vi "DSF Mini Explorer.vi"(7 "Item Type":T1=enum."Setting", 8 "error in (no error)":errorcluster, 10 "Item ID":string, 11 "explorer data":T2) -> (0 "error out":errorcluster)   [LabVIEW 2017, in "DSF Mini Explorer.lvlib"]
uses:
  DSF Mini Explorer.lvlib
  Main VI/Application Data.ctl
  VeriStand/Data Sharing Custom Device/Source/DSF Core.lvlibp/Classes/Configuration/Configuration Session.lvclass
  Main VI/View Mode.ctl
  Item Tree/ID to Tree Items/Tree Item Type.ctl
  Item Tree/Create New Tree Item.vi
  VeriStand/Data Sharing Custom Device/Source/DSF Core.lvlibp/Classes/Configuration/Remove ID.vi
  VeriStand/Data Sharing Custom Device/Source/DSF Core.lvlibp/Classes/Configuration/Read Item.vi
  VeriStand/Data Sharing Custom Device/Source/DSF Core.lvlibp/Classes/Configuration/Read Plugin.vi
  VeriStand/Data Sharing Custom Device/Source/DSF Core.lvlibp/Classes/Configuration/Read Settings.vi
  VeriStand/Data Sharing Custom Device/Source/DSF Core.lvlibp/Classes/Configuration/Read Group.vi
  VeriStand/Data Sharing Custom Device/Source/DSF Core.lvlibp/Classes/Configuration/Read Transfer.vi
  VeriStand/Data Sharing Custom Device/Source/DSF Core.lvlibp/Classes/Configuration/Read Channel.vi
panel:
  in  "Item Tree":string(tree)
  in  "Value Tree":string(tree)
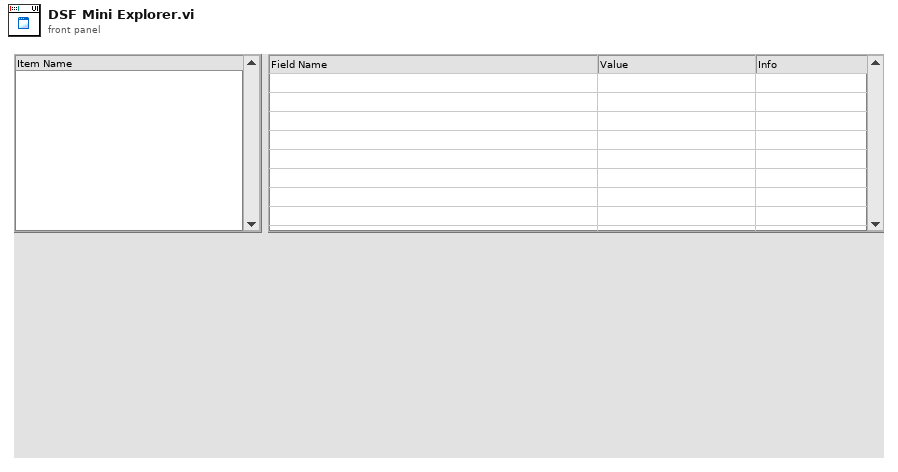
[diagram p1: front panel]
types:
  T1 = typedef "DSF Mini Explorer.lvlib/Tree Item Type.ctl" = enum16{"Plugin", "Group", "Transfer", "Channel", "Setting"}
  T2 = typedef "DSF Mini Explorer.lvlib/Application Data.ctl" = cluster{"Item Tree Control":refnum<vi>, "Value Tree Control":refnum<vi>, "DSF Refnum":refnum<class "Configuration Session.lvclass">, "Top-Level VI":refnum<vi>, "View State":T3}
  T3 = typedef "DSF Mini Explorer.lvlib/View Mode.ctl" = enum16{"Tree", "List"}
  T4 = typedef "DSF Mini Explorer.lvlib/Tree Item.ctl" = cluster{"Left Cell String":string, "Child Text":string[], "Child Tag":string, "Glyph Index":i32}
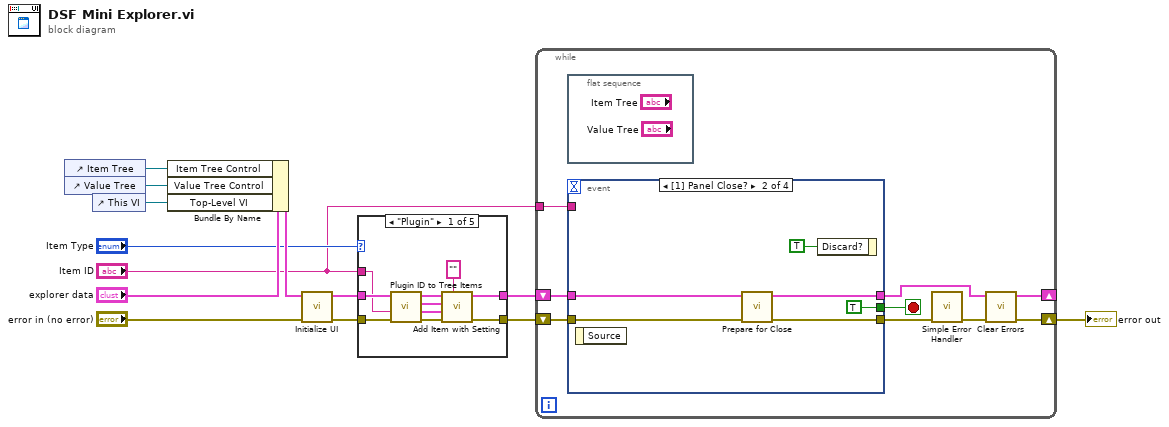
[diagram p0: block diagram]
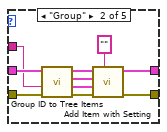
[diagram p2: hidden frame]
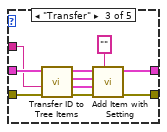
[diagram p3: hidden frame]
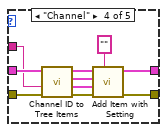
[diagram p4: hidden frame]
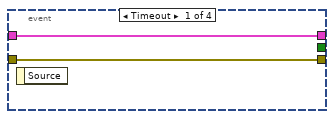
[diagram p6: hidden frame]
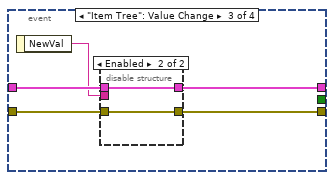
[diagram p7: hidden frame]
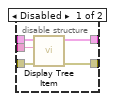
[diagram p8: hidden frame]
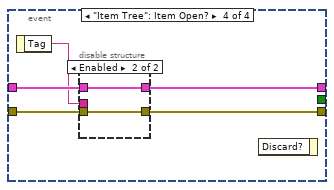
[diagram p9: hidden frame]
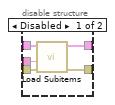
[diagram p10: hidden frame]
diagram:
  n1 = control-ref of="Item Tree"() -> (w9:refnum<vi>)
  n2 = control-ref of="Value Tree"() -> (w10:refnum<vi>)
  n3 = control-ref of="This VI"() -> (w2:refnum<vi>)
  n4 = Bundle By Name(cluster="explorer data", "Item Tree Control"=w9, "Value Tree Control"=w10, "Top-Level VI"=w2) -> (w12:T2)
  n5 = call "Initialize UI.vi"("error in (no error)"="error in (no error)", "Application Data in"=w12) -> ("error out"=w6:errorcluster, "Application Data out"=w7:T2)  [unwired: 8 in]
  n6 = case shown="\"Plugin\"" "Item Type" {
    tunnel: w7 -> [w23 w29 w40 w47 w55]
    tunnel: w6 -> [w22 w30 w38 w48 w54]
    tunnel: [w17 w32 w42 w52 w54] -> w5
    tunnel: [w18 w33 w43 w53 w55] -> w4
    tunnel: "Item ID" -> [w21 w24 w37 w46 _]
    frame "Plugin" {
      n7 = call "Plugin ID to Tree Items.vi"("error in (no error)"=w22, "Plugin ID"=w21, "Application Data in"=w23) -> ("error out"=w19:errorcluster, "Settings"=w15:T4, "Item"=w16:T4, "Application Data out"=w20:T2)  [unwired: 5 in]
      n8 = call "Add Item with Setting.vi"("Parent Tag"="", "error in (no error)"=w19, "Setting"=w15, "Item"=w16, "Application Data in"=w20) -> ("error out"=w17:errorcluster, "Application Data out"=w18:T2)  [unwired: 4 in, 1 out]
    }
    frame "Group" {
      n9 = call "Group ID to Tree Items.vi"("error in (no error)"=w30, "Group ID"=w24, "Application Data in"=w29) -> ("error out"=w27:errorcluster, "Settings"=w25:T4, "Item"=w26:T4, "Application Data out"=w28:T2)  [unwired: 5 in]
      n10 = call "Add Item with Setting.vi"("Parent Tag"="", "error in (no error)"=w27, "Setting"=w25, "Item"=w26, "Application Data in"=w28) -> ("error out"=w32:errorcluster, "Application Data out"=w33:T2)  [unwired: 4 in, 1 out]
    }
    frame "Transfer" {
      n11 = call "Transfer ID to Tree Items.vi"("error in (no error)"=w38, "Transfer ID"=w37, "Application Data in"=w40) -> ("error out"=w36:errorcluster, "Settings"=w35:T4, "Item"=w34:T4, "Application Data out"=w39:T2)  [unwired: 5 in]
      n12 = call "Add Item with Setting.vi"("Parent Tag"="", "error in (no error)"=w36, "Setting"=w35, "Item"=w34, "Application Data in"=w39) -> ("error out"=w42:errorcluster, "Application Data out"=w43:T2)  [unwired: 4 in, 1 out]
    }
    frame "Channel" {
      n13 = call "Channel ID to Tree Items.vi"("error in (no error)"=w48, "Channel ID"=w46, "Application Data in"=w47) -> ("error out"=w49:errorcluster, "Settings"=w44:T4, "Item"=w45:T4, "Application Data out"=w50:T2)  [unwired: 5 in]
      n14 = call "Add Item with Setting.vi"("Parent Tag"="", "error in (no error)"=w49, "Setting"=w44, "Item"=w45, "Application Data in"=w50) -> ("error out"=w52:errorcluster, "Application Data out"=w53:T2)  [unwired: 4 in, 1 out]
    }
    frame "Setting" {
    }
  }
  n15 = while {
    shift-right: [w57] -> w13
    shift-left: w5 -> [w62]
    shift-right: [w58] -> _
    shift-left: w4 -> [w59]
    tunnel: "Item ID" -> [w56]
    stop <- w63 stop-if-true
    n16 = flat-sequence {
      frame #0 {
      }
    }
    n17 = event shown="[1] Panel Close?" {
      selector: _ -> [_ _ _ _]
      dyn-events: _ -> [_ _ _ _]
      timeout: _ -> [_ _ _ _]
      tunnel: [_ TRUE _ _] -> w63
      tunnel: w62 -> [w65 w70 w76 w88]
      tunnel: [w65 w67 w75 w87] -> w60
      tunnel: w59 -> [w64 w68 w73 w86]
      tunnel: [w64 w66 w74 w85] -> w58
      tunnel: w56 -> [_ _ _ _]
      event Timeout {
        n18 = event-data() -> ()  [unwired: 1 in, 1 out]
      }
      event Panel Close? {
        n19 = event-data() -> ()  [unwired: 1 in, 1 out]
        n20 = call "Prepare for Close.vi"("error in (no error)"=w70, "Application Data in"=w68) -> ("error out"=w67:errorcluster, "Application Data out"=w66:T2)  [unwired: 8 in]
        n21 = event-data("Discard?"=TRUE) -> ()  [unwired: 1 in, 1 out]
      }
      event "Item Tree": Value Change {
        n22 = event-data() -> ("NewVal"=w72:string)  [unwired: 1 in]
        n23 = disable-structure shown="Enabled" {
          disable-tunnel: w76 -> [w81 w82]
          disable-tunnel: [w80 w82] -> w75
          disable-tunnel: [w79 w83] -> w74
          disable-tunnel: w73 -> [w78 w83]
          disable-tunnel: w72 -> [w77 _]
          frame Disabled {
            n24 = call "Display Tree Item.vi"("error in (no error)"=w81, "Tag"=w77, "Application Data in"=w78) -> ("error out"=w80:errorcluster, "Application Data out"=w79:T2)  [unwired: 7 in]
          }
          frame Enabled {
          }
        }
      }
      event "Item Tree": Item Open? {
        n25 = event-data() -> ("Tag"=w84:string)  [unwired: 1 in]
        n26 = disable-structure shown="Enabled" {
          disable-tunnel: w88 -> [w93 w94]
          disable-tunnel: [w92 w94] -> w87
          disable-tunnel: w86 -> [w91 w95]
          disable-tunnel: [w90 w95] -> w85
          disable-tunnel: w84 -> [w89 _]
          frame Disabled {
            n27 = call "Load Subitems.vi"("error in (no error)"=w93, "Tag"=w89, "Application Data in"=w91) -> ("error out"=w92:errorcluster, "Application Data out"=w90:T2)  [unwired: 6 in, 1 out]
          }
          frame Enabled {
          }
        }
        n28 = event-data() -> ()  [unwired: 2 in, 1 out]
      }
    }
    n29 = call <vilib>:"Simple Error Handler.vi"("error in (no error)"=w60) -> ("error out"=w61:errorcluster)  [unwired: 4 in, 4 out]
    n30 = call <vilib>:"Clear Errors.vi"("error in (no error)"=w61) -> ("error out"=w57:errorcluster)  [unwired: 5 in, 1 out]
  }
  "error out" <- w13
